vi "Arduino generic wrapper.vi"(2 "Tx msg cluster":T1={"dest"=1, "A/D/C/I"="A", "R/W"="R", "chan"=1, "val (float)"=0.0}, 3 "Channel Name":string, 4 "Port name":string) -> (0 "Scan comment":string, 1 "Output":dbl)   [LabVIEW 2018]
uses:
  ctls_and_globals/Arduino tx msg cluster.ctl
  ctls_and_globals/Arduino Config & resource typedef.ctl
  ctls_and_globals/Arduino Global.vi
panel:
  out "error out":errorcluster
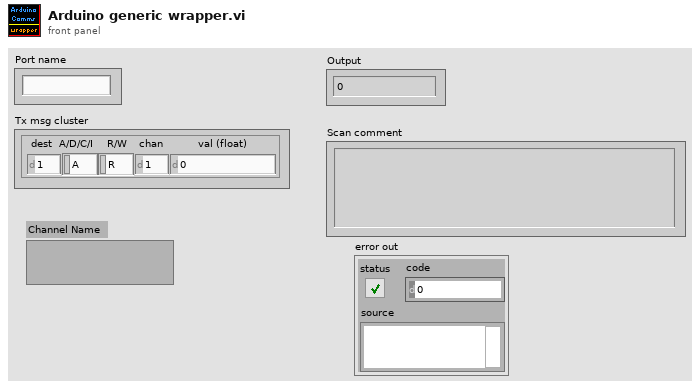
[diagram p1: front panel]
types:
  T1 = typedef "Arduino tx msg cluster.ctl" = cluster{"dest":u8, "A/D/C/I":string, "R/W":string, "chan":u8, "val (float)":sgl}
  T2 = typedef "Arduino Config & resource typedef.ctl" = cluster{"baud rate (bps)":u32, "timeout (ms)":u32, "data bits":u16, "parity":enum16{"None", "Odd", "Even", "Mark", "Space"}, "stop bits (10: 1 bit)":u16, "flow control":u16, "termination char (hex)":u8, "Enable Termination Char":bool, "byte count":u32, "Resource locked?":bool}
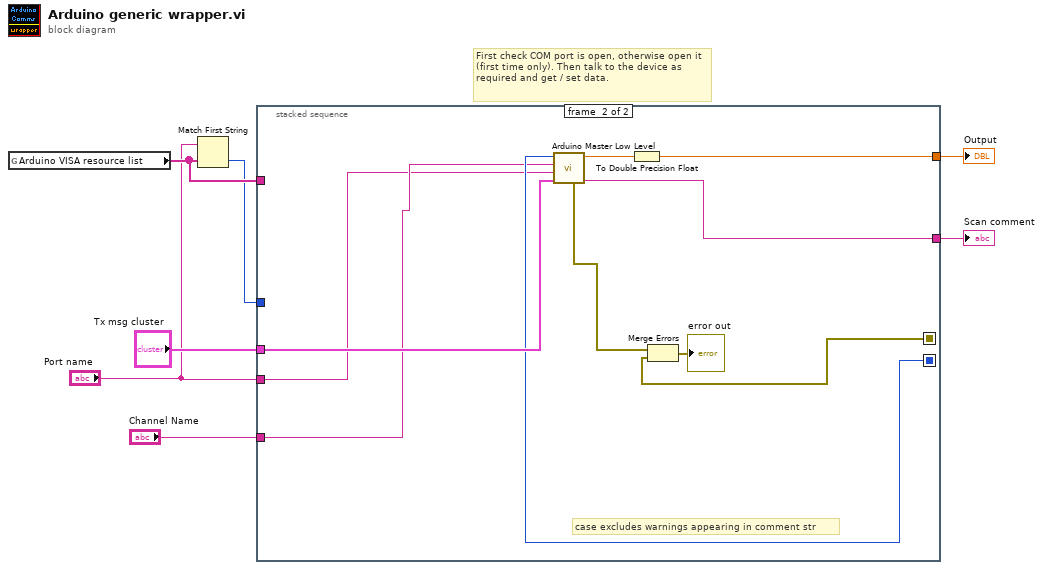
[diagram p0: block diagram]
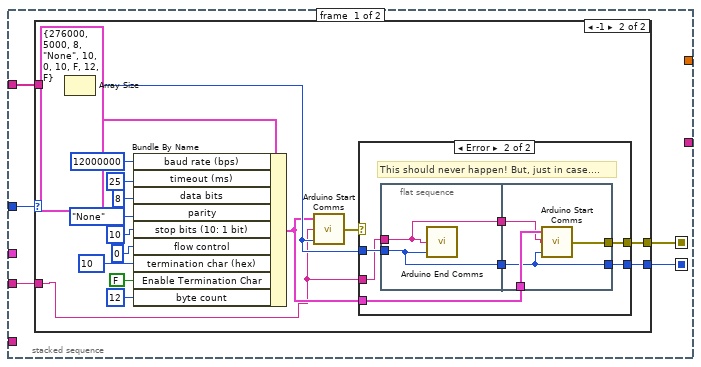
[diagram p2: hidden frame]
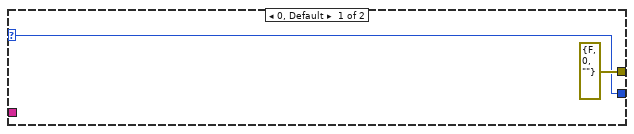
[diagram p3: hidden frame]
diagram:
  # "First check COM port is open, otherwise open it (first time only). Then talk to the device as required and get / set data."
  n1 = global read "Arduino Global.vi" "Arduino VISA resource list"() -> (w7:string[])
  n2 = Match First String(2:w7, 3:"Port name") -> (0:w6:i32)  [unwired: 1 out]
  n3 = stacked-sequence {
    seq-local: [w9 _] -> [_ w50]
    seq-local: [w8 _] -> [_ w53]
    tunnel: w6 -> [w12 _]
    tunnel: w7 -> [w11 _]
    tunnel: "Port name" -> [w10 w47]
    tunnel: [_ w55] -> w5
    tunnel: "Tx msg cluster" -> [_ w54]
    tunnel: [_ w48] -> w2
    tunnel: "Channel Name" -> [_ w52]
    frame #0 {
      n4 = case shown="-1" w12 {
        selector: w12 -> [w13 _]
        tunnel: w11 -> [_ w31]
        tunnel: w10 -> [_ w15]
        tunnel: [errorcluster {"status"=FALSE, "code"=0, "source"=""} ("Error") w17] -> w9
        tunnel: [w13 w16] -> w8
        frame 0, Default {
        }
        frame -1 {
          n5 = Array Size(array=w31) -> (size(s)=w19:i32)
          n6 = Bundle By Name(cluster=T2 {"baud rate (bps)"=276000, "timeout (ms)"=5000, "data bits"=8, "parity"=enum."None", "stop bits (10: 1 bit)"=10, "flow control"=0, "termination char (hex)"=10, "Enable Termination Char"=FALSE, "byte count"=12, "Resource locked?"=FALSE} ("Arduino VISA config & resource"), "baud rate (bps)"=u32 12000000, "timeout (ms)"=u32 25, "data bits"=u16 8, "parity"=enum16{"None", "Odd", "Even", "Mark", "Space"}."None", "stop bits (10: 1 bit)"=u16 10, "flow control"=u16 0, "termination char (hex)"=u8 10, "Enable Termination Char"=FALSE, "byte count"=u32 12) -> (w18:T2)
          n7 = call "Arduino Start Comms.vi"("Resource index"=w19, "VISA resource name"=w15, "Arduino VISA config & resource"=w18) -> ("Error"=w20:errorcluster)
          n8 = case shown="Error" w20 {
            selector: w20 -> [w33 _]
            tunnel: w19 -> [w32 w40]
            tunnel: w18 -> [_ w39]
            tunnel: [w33 w37] -> w17
            tunnel: [w32 w36] -> w16
            tunnel: w15 -> [_ w35]
            frame No Error {
            }
            frame Error {
              # "This should never happen! But, just in case...."
              n9 = flat-sequence {
                tunnel: w40 -> [w42]
                tunnel: [w42] -> w38
                tunnel: w35 -> [w41]
                tunnel: [w41] -> w34
                tunnel: w39 -> [w46]
                tunnel: w38 -> [w44]
                tunnel: [w45] -> w37
                tunnel: [w44] -> w36
                tunnel: w34 -> [w43]
                frame #0 {
                  n10 = call "Arduino End Comms.vi"("Resource index"=w42, "VISA resource name"=w41) -> ()  [unwired: 2 out]
                }
                frame #1 {
                  n11 = call "Arduino Start Comms.vi"("Resource index"=w44, "VISA resource name"=w43, "Arduino VISA config & resource"=w46) -> ("Error"=w45:errorcluster)
                }
              }
            }
          }
        }
      }
    }
    frame #1 {
      # "case excludes warnings appearing in comment str"
      n12 = call "Arduino Master Low Level.vi"("Arduino VISA resource index"=w53, "Channel Name"=w52, "VISA resource name"=w47, "Tx msg cluster"=w54) -> ("Error"=w51:errorcluster, "Value returned"=w56:sgl, "Scan Comments"=w48:string)  [unwired: 2 out]
      n13 = To Double Precision Float(number=w56) -> (double precision float=w55:dbl)
      n14 = Merge Errors(w51, w50) -> (→"error out":errorcluster)
    }
  }
  "Output" <- w5
  "Scan comment" <- w2
